vi "Lab16_genSub.vi"(5 "duty cycle":dbl=0.5 format="%.6f", 7 "frequency":dbl=1.0 format="%.6f", 8 "error in":errorcluster, 10 "CO.Pulse.Term":tag="/Dev1/PFI1", 11 "task in":refnum<k21>) -> (0 "error out":errorcluster, 3 "task out":refnum<k21>)   [LabVIEW 2022 SP3]
uses:
  <vilib>/DAQmx/configure/timing.llb/DAQmx Timing (Implicit).vi
  <resource>/objmgr/daqmx.rc
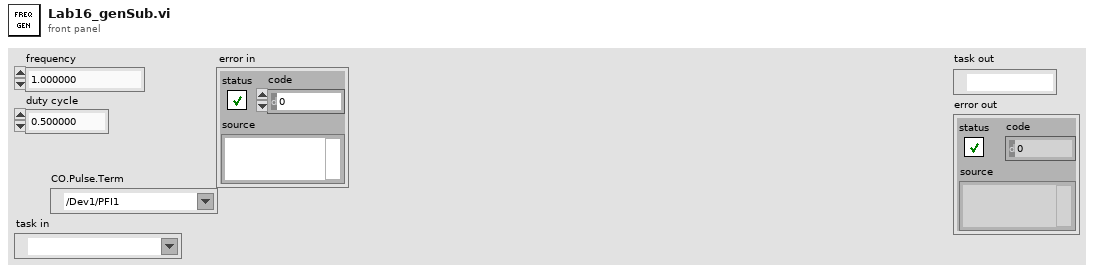
[diagram p1: front panel]
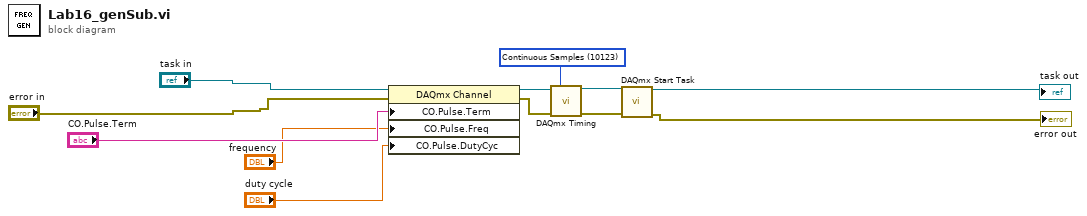
[diagram p0: block diagram]
diagram:
  w12 = 10123 items=["Finite Samples"=10178, "Continuous Samples"=10123, "Hardware Timed Single Point"=12522] ("sample mode")
  n1 = property class="DAQmx Channel"(reference="task in", error in="error in", "CO.Pulse.Term"="CO.Pulse.Term", "CO.Pulse.Freq"="frequency", "CO.Pulse.DutyCyc"="duty cycle") -> (reference out=w8:refnum<k21>, error out=w9:errorcluster)
  n2 = call-poly <vilib>:"DAQmx Timing.vi"("task/channels in"=w8, "sample mode"=w12, "error in"=w9) -> ("task out"=w10:refnum<k21>, "error out"=w11:errorcluster)  [unwired: 11 in]
  n3 = call <vilib>:"DAQmx Start Task.vi"("task/channels in"=w10, "error in"=w11) -> ("task out"=→"task out":refnum<k21>, "error out"=→"error out":errorcluster)  [unwired: 12 in]
